vi "Yokogawa GS200 Initialize.vi"(3 "Error In":errorcluster, 6 "VISA resource name":refnum<visa-resource-name>) -> (0 "Error Out":errorcluster, 1 "Instrument ID String":string, 2 "dup VISA Session":refnum<visa-resource-name>)   [LabVIEW 2021]
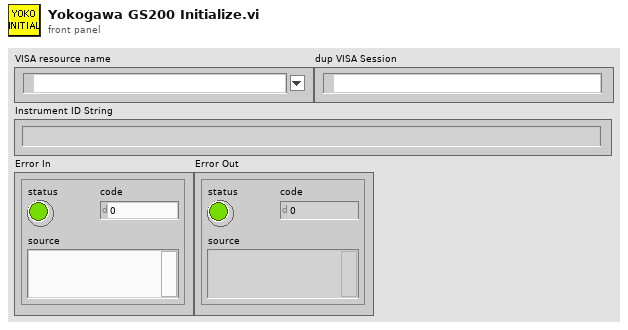
[diagram p1: front panel]
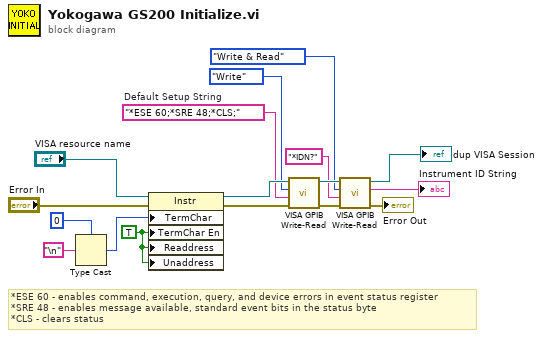
[diagram p0: block diagram]
diagram:
  w2 = "*ESE 60;*SRE 48;*CLS;"  # Default Setup String
  w10 = TRUE
  # "*ESE 60 - enables command, execution, query, and device errors in event status register\n*SRE 48 - enables message available, standard event bits in the status byte\n*CLS - clears status"
  n1 = Type Cast(type=u8 0 ("Message Based Settings:Termination Character"), x="\n") -> (*(type *) &x=w14:u8)
  n2 = property class="Instr"(reference="VISA resource name", error in="Error In", "TermChar"=w14, "TermChar En"=w10, "Readdress"=w10, "Unaddress"=w10) -> (reference out=w16:refnum<visa-resource-name>, error out=w12:errorcluster)
  n3 = call "VISA GPIB Write-Read.vi"("error in (no error)"=w12, "Command"=w2, "Action"=enum16{"Write", "Read", "Write & Read"}."Write", "VISA resource name"=w16) -> ("error out"=w8:errorcluster, "dup VISA Session"=w9:refnum<visa-resource-name>)  [unwired: 4 in, 2 out]
  n4 = call "VISA GPIB Write-Read.vi"("error in (no error)"=w8, "Command"="*IDN?", "Action"=enum16{"Write", "Read", "Write & Read"}."Write & Read", "VISA resource name"=w9) -> ("error out"=→"Error Out":errorcluster, "String Returned"=→"Instrument ID String":string, "dup VISA Session"=→"dup VISA Session":refnum<visa-resource-name>)  [unwired: 4 in, 1 out]
